vi "vCone unit converter.vi"(8 "temp (C)":dbl, 9 "deltaP (Pa)":dbl, 10 "staticP (Pa Gauge)":dbl, 11 "ambientP (Pa)":dbl) -> (3 "mDot":dbl caption="massFlow (kg/s)")   [LabVIEW 2018]
uses:
  Chris VIs/V-cone/V-Cone CompressorRig.vi
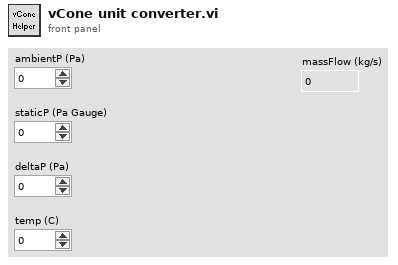
[diagram p1: front panel]
types:
  T1 = cluster{"delta P (mBar)":dbl, "T (K)":dbl, "Upstream (barA)":dbl}
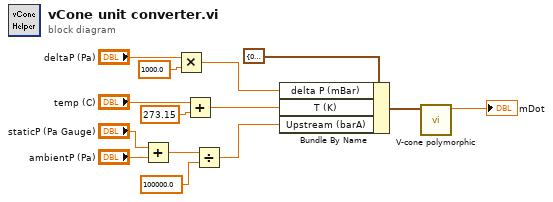
[diagram p0: block diagram]
diagram:
  n1 = Add(x="staticP (Pa Gauge)", y="ambientP (Pa)") -> (x+y=w12:dbl)
  n2 = Multiply(x="deltaP (Pa)", y=1000.0) -> (x*y=w6:dbl)
  n3 = Add(x="temp (C)", y=273.15) -> (x+y=w9:dbl)
  n4 = Divide(x=w12, y=100000.0) -> (x/y=w13:dbl)
  n5 = Bundle By Name(cluster=T1 {"delta P (mBar)"=0.0, "T (K)"=0.0, "Upstream (barA)"=0.0} ("Measurements"), "delta P (mBar)"=w6, "T (K)"=w9, "Upstream (barA)"=w13) -> (w3:T1)
  n6 = call-poly "V-cone polymorphic.vi"("Measurements"=w3) -> ("Mass Flowrate (Kg/s)"=→"mDot":dbl)  [unwired: 9 in, 1 out]
